vi "WAV_Binarize.vi"(10 "Data in":sgl[][](graph), 11 "format":T1) -> (2 "file string":string)   [LabVIEW 2022 SP3]
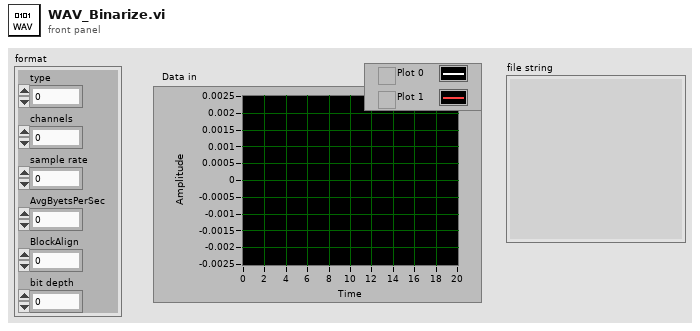
[diagram p1: front panel]
types:
  T1 = cluster{"type":u16, "channels":u16, "sample rate":u32, "AvgByetsPerSec":u32, "BlockAlign":u16, "bit depth":u16}
  T2 = enum16{"big-endian, network order", "native, host order", "little-endian"}
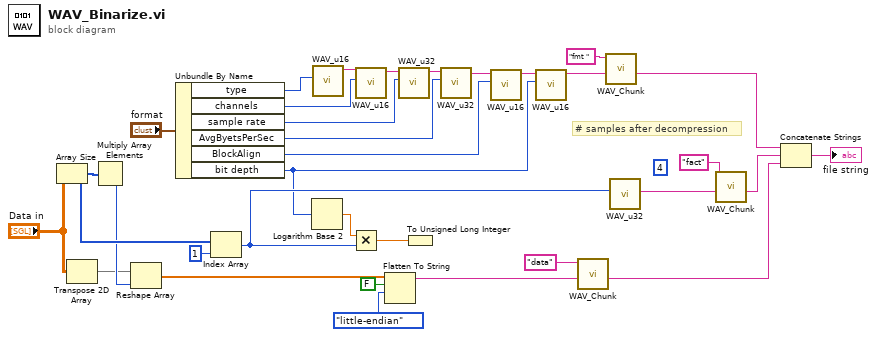
[diagram p0: block diagram]
diagram:
  (unwired) u32 4 ("u32")
  # "# samples after decompression"
  n1 = Array Size(array="Data in") -> (size(s)=w18:i32[])
  n2 = Transpose 2D Array(2D array="Data in") -> (transposed array=w12:sgl[][])
  n3 = Multiply Array Elements(1:w18) -> (0:w14:i32)
  n4 = Reshape Array(w12, w14) -> (w21:sgl[])
  n5 = Unbundle By Name("format") -> ("type"=w24:u16, "channels"=w26:u16, "sample rate"=w31:u32, "AvgByetsPerSec"=w23:u32, "BlockAlign"=w30:u16, "bit depth"=w10:u16)
  n6 = Index Array(array=w18, index=1) -> (element=w32:i32)
  n7 = Logarithm Base 2(1:w10) -> (0:w9:dbl)
  n8 = call "WAV_u16.vi"("u16"=w24) -> ("String out"=w25:string)  [unwired: 10 in]
  n9 = Multiply(x=w9, y=w32) -> (x*y=w33:dbl)
  n10 = call "WAV_u16.vi"("u16"=w26, "String in"=w25) -> ("String out"=w27:string)  [unwired: 9 in]
  n11 = Flatten To String(anything=w21, prepend array or string size? (T)=FALSE, byte order (0:big-endian, network order)=T2."little-endian") -> (data string=w8:string)  [unwired: 1 in, 2 out]
  n12 = call "WAV_u32.vi"("u32"=w31, "String in"=w27) -> ("String out"=w22:string)  [unwired: 9 in]
  n13 = To Unsigned Long Integer(number=w33) -> ()  [unwired: 1 out]
  n14 = call "WAV_u32.vi"("u32"=w23, "String in"=w22) -> ("String out"=w29:string)  [unwired: 9 in]
  n15 = call "WAV_u16.vi"("u16"=w30, "String in"=w29) -> ("String out"=w28:string)  [unwired: 9 in]
  n16 = call "WAV_u16.vi"("u16"=w10, "String in"=w28) -> ("String out"=w4:string)  [unwired: 9 in]
  n17 = call "WAV_Chunk.vi"("data string"=w8, "string"="data") -> ("String out"=w7:string)  [unwired: 9 in]
  n18 = call "WAV_Chunk.vi"("data string"=w4, "string"="fmt ") -> ("String out"=w5:string)  [unwired: 9 in]
  n19 = call "WAV_u32.vi"("u32"=w32) -> ("String out"=w3:string)  [unwired: 10 in]
  n20 = call "WAV_Chunk.vi"("data string"=w3, "string"="fact" ("String")) -> ("String out"=w1:string)  [unwired: 9 in]
  n21 = Concatenate Strings(w5, w1, w7) -> (→"file string":string)
